vi "GUI_CH1_Comm_TCPIP_NEW.vi"() -> ()   [LabVIEW 2018]
uses:
  RxTx/RxTx.lvclass
  TCPIP/TCPIP.lvclass
panel:
  in  "Remote port ACS":u16=59041
  in  "stop":bool
  out "error out 5":errorcluster
  out "error out 4":errorcluster
  out "error out 3":errorcluster
  in  "IP":string="200.131.64.49"
  in  "TCPIP.lvclass 3":refnum<class "TCPIP.lvclass">
  out "error out 2":errorcluster
  in  "TCPIP.lvclass 2":refnum<class "TCPIP.lvclass">
  in  "RxTx.lvclass 2":refnum<class "RxTx.lvclass">
  in  "Channel":u16=1
  in  "Remote port GUI":u16=54165
  # "Channel 1 - TCPIP Communication"
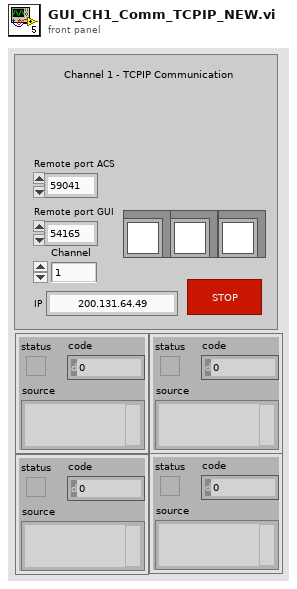
[diagram p1: front panel]
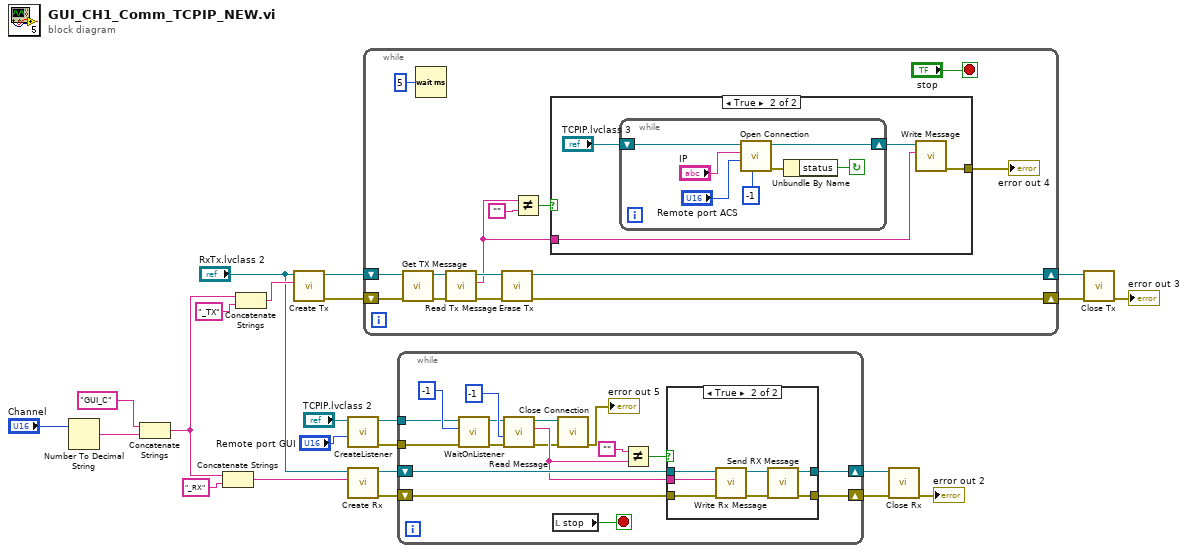
[diagram p0: block diagram]
diagram:
  n1 = Number To Decimal String(number="Channel") -> (decimal integer string=w20:string)  [unwired: 1 in]
  n2 = Concatenate Strings("GUI_C", w20) -> (w7:string)
  n3 = Concatenate Strings(w7, "_RX" ("Reader Name")) -> (w23:string)
  n4 = Concatenate Strings(w7, "_TX" ("Reader Name")) -> (w11:string)
  n5 = call "Create Tx.vi"("Writer Name"=w11, "RxTx in"="RxTx.lvclass 2") -> ("error out"=w8:errorcluster, "RxTx out"=w9:refnum<class "RxTx.lvclass">)  [unwired: 8 in]
  n6 = call-dynamic "CreateListener.vi"("remote port"="Remote port GUI", "TCPIP in"="TCPIP.lvclass 2") -> ("error out"=w12:errorcluster, "TCPIP out"=w16:refnum<class "TCPIP.lvclass">)  [unwired: 8 in]
  n7 = call "Create Rx.vi"("Reader Name"=w23, "RxTx in"="RxTx.lvclass 2") -> ("error out"=w17:errorcluster, "RxTx out"=w18:refnum<class "RxTx.lvclass">)  [unwired: 8 in]
  n8 = while {
    shift-right: [w37] -> w6
    shift-left: w9 -> [w30]
    shift-right: [w36] -> w5
    shift-left: w8 -> [w29]
    stop <- "stop" stop-if-true
    n9 = call "Get TX Message.vi"("error in (no error)"=w29, "RxTx in"=w30) -> ("error out"=w35:errorcluster, "RxTx out"=w31:refnum<class "RxTx.lvclass">)  [unwired: 8 in]
    n10 = Wait (ms)(milliseconds to wait=u32 5) -> ()  [unwired: 1 out]
    n11 = call "Read Tx Message.vi"("error in (no error)"=w35, "RxTx in"=w31) -> ("error out"=w32:errorcluster, "Tx Message"=w27:string, "RxTx out"=w33:refnum<class "RxTx.lvclass">)  [unwired: 7 in]
    n12 = call "Erase Tx.vi"("error in (no error)"=w32, "RxTx in"=w33) -> ("error out"=w36:errorcluster, "RxTx out"=w37:refnum<class "RxTx.lvclass">)  [unwired: 8 in]
    n13 = Not Equal?(x=w27, y="") -> (x != y?=w28:bool)
    n14 = case shown="True" w28 {
      tunnel: w27 -> [_ w39]
      tunnel: [_ w38] -> w26
      frame False {
      }
      frame True {
        n15 = while {
          shift-right: [w47] -> w41
          shift-left: "TCPIP.lvclass 3" -> [w48]
          stop <- w45 continue-if-true
          n16 = call "Open Connection.vi"("timeout"=-1, "remote port"="Remote port ACS", "IP"="IP", "TCPIP in"=w48) -> ("error out"=w43:errorcluster, "TCPIP out"=w47:refnum<class "TCPIP.lvclass">)  [unwired: 6 in]
          n17 = Unbundle By Name(w43) -> ("status"=w45:bool)
        }
        n18 = call "Write Message.vi"("Message"=w39, "TCPIP in"=w41) -> ("error out"=w38:errorcluster)  [unwired: 8 in, 1 out]
      }
    }
    "error out 4" <- w26
  }
  n19 = while {
    shift-right: [w56] -> w14
    shift-left: w17 -> [w65]
    shift-right: [w57] -> w15
    shift-left: w18 -> [w64]
    tunnel: w16 -> [w54]
    tunnel: w12 -> [w51]
    stop <- w49 stop-if-true
    n20 = call-dynamic "WaitOnListener.vi"("error in (no error)"=w51, "timeout ms"=-1, "TCPIP in"=w54) -> ("error out"=w58:errorcluster, "TCPIP out"=w59:refnum<class "TCPIP.lvclass">)  [unwired: 7 in]
    n21 = call "Read Message.vi"("error in (no error)"=w58, "timeout"=-1, "TCPIP in"=w59) -> ("error out"=w53:errorcluster, "Message"=w60:string, "TCPIP out"=w52:refnum<class "TCPIP.lvclass">)  [unwired: 6 in]
    n22 = local read "stop"() -> (w49:bool)
    n23 = call "Close Connection.vi"("error in (no error)"=w53, "TCPIP in"=w52) -> ("error out"=→"error out 5":errorcluster)  [unwired: 8 in, 1 out]
    n24 = Not Equal?(x="", y=w60) -> (x != y?=w62:bool)
    n25 = case shown="True" w62 {
      tunnel: w65 -> [w66 w72]
      tunnel: w64 -> [w67 w71]
      tunnel: [w67 w69] -> w57
      tunnel: [w66 w68] -> w56
      tunnel: w60 -> [_ w70]
      frame False {
      }
      frame True {
        n26 = call "Write Rx Message.vi"("error in (no error)"=w72, "Rx Message"=w70, "RxTx in"=w71) -> ("error out"=w73:errorcluster, "RxTx out"=w74:refnum<class "RxTx.lvclass">)  [unwired: 7 in]
        n27 = call "Send RX Message.vi"("error in (no error)"=w73, "RxTx in"=w74) -> ("error out"=w68:errorcluster, "RxTx out"=w69:refnum<class "RxTx.lvclass">)  [unwired: 8 in]
      }
    }
  }
  n28 = call "Close Rx.vi"("error in (no error)"=w14, "RxTx in"=w15) -> ("error out"=→"error out 2":errorcluster)  [unwired: 8 in, 1 out]
  n29 = call "Close Tx.vi"("error in (no error)"=w5, "RxTx in"=w6) -> ("error out"=→"error out 3":errorcluster)  [unwired: 8 in, 1 out]
